vi "表格初始化.vi"(0 "表格引用":refnum<vi>, 5 "索引":i32, 7 "长度":i32, 11 "错误输入（无错误）":errorcluster) -> (4 "引用输出":refnum<vi>, 6 "行首字符串[]":string[](array[string]), 8 "列首字符串[]":string[](array[string]), 10 "文本数据":string[][](array[string]), 15 "错误输出":errorcluster)   [LabVIEW 2018]
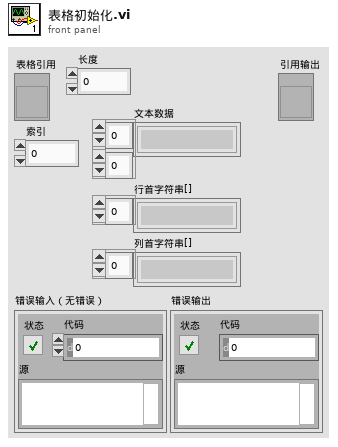
[diagram p1: front panel]
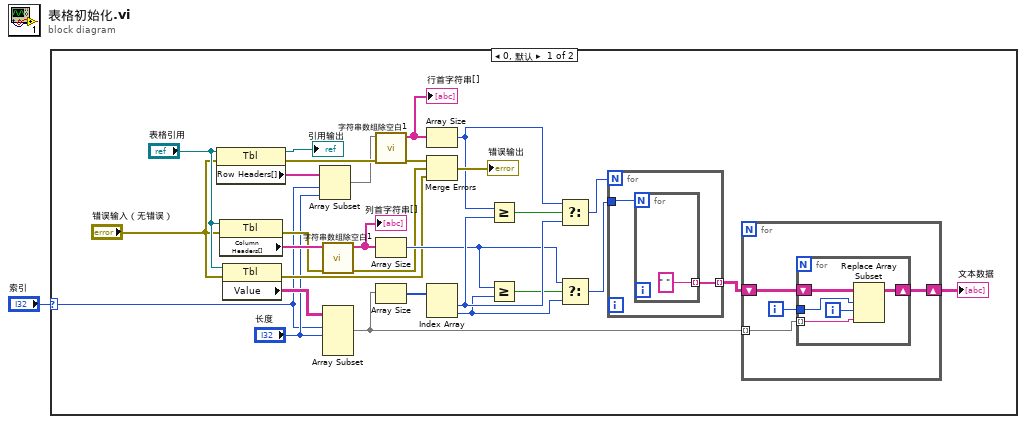
[diagram p0: block diagram]
diagram:
  n1 = case shown="0, 默认" "索引" {
    selector: "索引" -> [w2 _]
    frame 0, Default {
      n2 = property class="Tbl"(reference="表格引用", error in="错误输入（无错误）") -> (reference out=→"引用输出":refnum<vi>, error out=w12:errorcluster, "Row Headers[]"=w7:string[])
      n3 = property class="Tbl"(reference="表格引用", error in="错误输入（无错误）") -> (error out=w10:errorcluster, "Column Headers[]"=w14:string[])  [unwired: 1 out]
      n4 = property class="Tbl"(reference="表格引用", error in="错误输入（无错误）") -> (error out=w8:errorcluster, "Value"=w5:string[][])  [unwired: 1 out]
      n5 = Array Subset(array=w7, index=w2, length="长度") -> (w6:string[])
      n6 = call "字符串数组除空白1.vi"("error in (no error)"=w10, "输入字符串数组"=w14) -> ("错误输出"=w9:errorcluster, "输出字符串数组"=w13:string[])  [unwired: 8 in]
      "列首字符串[]" <- w13
      n7 = Array Subset(array=w5, index (row)=w2, length (row)="长度") -> (w4:string[][])  [unwired: 2 in]
      n8 = call "字符串数组除空白1.vi"("error in (no error)"=w12, "输入字符串数组"=w6) -> ("错误输出"=w11:errorcluster, "输出字符串数组"=w15:string[])  [unwired: 8 in]
      "行首字符串[]" <- w15
      n9 = Array Size(array=w13) -> (size(s)=w18:i32)
      n10 = Array Size(array=w4) -> (size(s)=w24:i32[])
      n11 = Array Size(array=w15) -> (size(s)=w23:i32)
      n12 = Merge Errors(w11, w9, w8) -> (→"错误输出":errorcluster)
      n13 = Index Array(array=w24) -> (element #1=w22:i32, element #2=w17:i32)  [unwired: 2 in]
      n14 = Greater Or Equal?(x=w23, y=w22) -> (x >= y?=w21:bool)
      n15 = Greater Or Equal?(x=w18, y=w17) -> (x >= y?=w19:bool)
      n16 = Select(t=w23, s=w21, f=w22) -> (s? t:f=w20:i32)
      n17 = Select(t=w18, s=w19, f=w17) -> (s? t:f=w16:i32)
      n18 = for {
        N: w20 -> [_]
        tunnel: w16 -> [w32]
        tunnel: [w31] -> w30 mode=indexing
        n19 = for {
          N: w32 -> [_]
          tunnel: [" "] -> w31 mode=indexing
        }
      }
      n20 = for {
        shift-right: [w36] -> w28
        shift-left: w30 -> [w37]
        tunnel: w4 -> [w34] mode=indexing
        i -> [w35]
        n21 = for {
          shift-right: [w41] -> w36
          shift-left: w37 -> [w42]
          tunnel: w35 -> [w39]
          tunnel: w34 -> [w40] mode=indexing
          i -> [w38]
          n22 = Replace Array Subset(array=w42, new element=w40, index (row)=w39, index (col)=w38) -> (w41:string[][])
        }
      }
      "文本数据" <- w28
    }
    frame -1 {
    }
  }
